vi "RootsPumpLCW_Main.vi"(7 "ref_stop_external":refnum<vi>, 8 "variable_reference":T1) -> ()   [LabVIEW 2019]
uses:
  cluster_ref_RootsPumpLCW.ctl
  <vilib>/MakerHub/LINX/LMH-LINX.lvlib
panel:
  out "time_now":dbl
  in  "Logging":bool=TRUE
  out "Logging Status":bool
  in  "Tab Control":enum32{"Flow Chart", "Raw Voltage Chart"}(tab)
  out "M1 Chart":waveform(dbl)[](graph)
  out "M2 Chart":waveform(dbl)[](graph)
  out "M3 Chart":waveform(dbl)[](graph)
  out "M4 Chart":waveform(dbl)[](graph)
  out "WFS1 Chart":waveform(dbl)[](graph)
  in  "SMS":bool=TRUE
  in  "M123_lo":dbl=0.3 caption="M1/M2/M3"
  in  "M123_lolo":dbl=0.2
  in  "WFS1_lo":dbl=1.3 caption="WFS1"
  in  "WFS1_lolo":dbl=1.2
  out "alarm_status":u32(colorbox) caption="Alarm Status"
  out "M1 Voltage Chart":waveform(dbl)[](graph)
  out "M2 Voltage Chart":waveform(dbl)[](graph)
  out "M3 Voltage Chart":waveform(dbl)[](graph)
  out "M4 Voltage Chart":waveform(dbl)[](graph)
  out "WFS1 Voltage Chart":waveform(dbl)[](graph)
  out "M1_V":dbl caption="V" format="%.2g"
  out "M4_V":dbl caption="V" format="%.2g"
  out "M3_V":dbl caption="V" format="%.2g"
  out "M2_V":dbl caption="V" format="%.2g"
  out "WFS1_V":dbl caption="V" format="%.2g"
  out "Meas. steps":i32
  in  "n_avg":i32=1000 caption="N of samples per meas."
  out "WFS1":dbl format="%.2g"
  in  "VISA":refnum<visa-resource-name>="COM25"
  out "M4":dbl format="%.2g"
  out "M3":dbl format="%.2g"
  in  "Meas. Interval":i32=30
  out "M2":dbl format="%.2g"
  out "M1":dbl format="%.2g"
  out "Readout Status":bool
  out "Last Measured":timestamp format="%<%Y-%m-%d %H:%M:%S>T"
  in  "Stop":bool
  # "Roots-Pump LCW Flow"
  # "sec"
  # "("
  # ")"
  # "("
  # ")"
  # "GPM"
  # "GPM"
  # "GPM"
  # "GPM"
  # "GPM"
  # "Warning:"
  # "GPM"
  # "Error:"
  # "GPM"
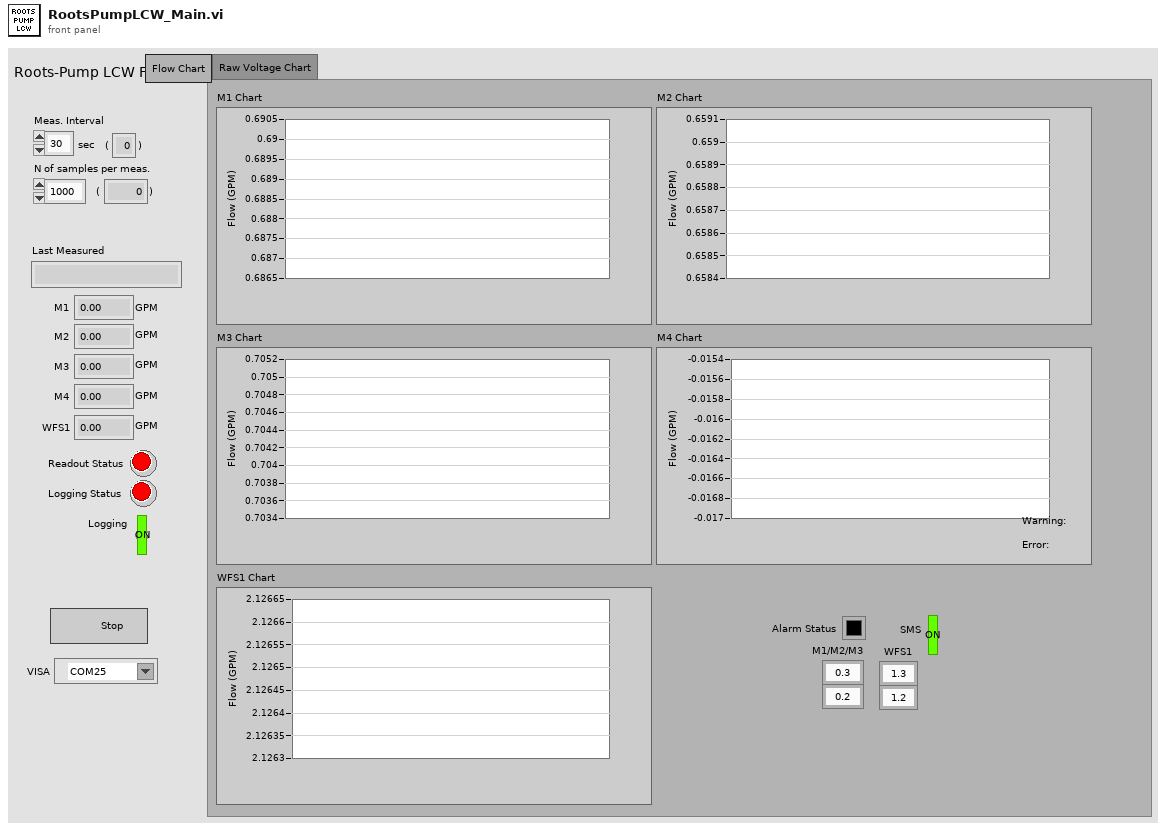
[diagram p1: front panel]
types:
  T1 = typedef "cluster_ref_RootsPumpLCW.ctl" = cluster{"Status":refnum<vi>, "M1":refnum<vi>, "M2":refnum<vi>, "M3":refnum<vi>, "M4":refnum<vi>, "WFS1":refnum<vi>}
  T2 = typedef "LMH-LINX.lvlib/LINX Ref.ctl" = cluster{"IO":T3, "Interface":T4, "LINX Device Config":T5}
  T3 = typedef "LMH-LINX.lvlib/Platform.ctl" = enum16{"Remote", "Local"}
  T4 = typedef "LMH-LINX.lvlib/Interface.ctl" = enum16{"Serial", "TCP"}
  T5 = typedef "LMH-LINX.lvlib/Device.lvlib/LINX Device Config.ctl" = cluster{"Interface":T4, "COM Port":refnum<visa-resource-name>, "TCP Configuration":T6, "Device Family":u8, "Device ID":u8, "Device Name":string, "TCP Ref":refnum<k5>, "Channels":T7}
  T6 = typedef "LMH-LINX.lvlib/Device.lvlib/TCP Config.ctl" = cluster{"IP Address":string, "Port":u16}
  T7 = typedef "LMH-LINX.lvlib/Channels.ctl" = cluster{"DI":u8[], "DO":u8[], "AI":u8[], "AO":u8[], "PWM":u8[], "QE":u8[], "UART":u8[], "I2C 2":u8[], "SPI":u8[], "CAN":u8[], "Servo":u8[], "AI Ref (V)":dbl, "AI Resolution (Bits)":u8, "AO Ref (V)":dbl, "AO Resolution (Bits)":u8}
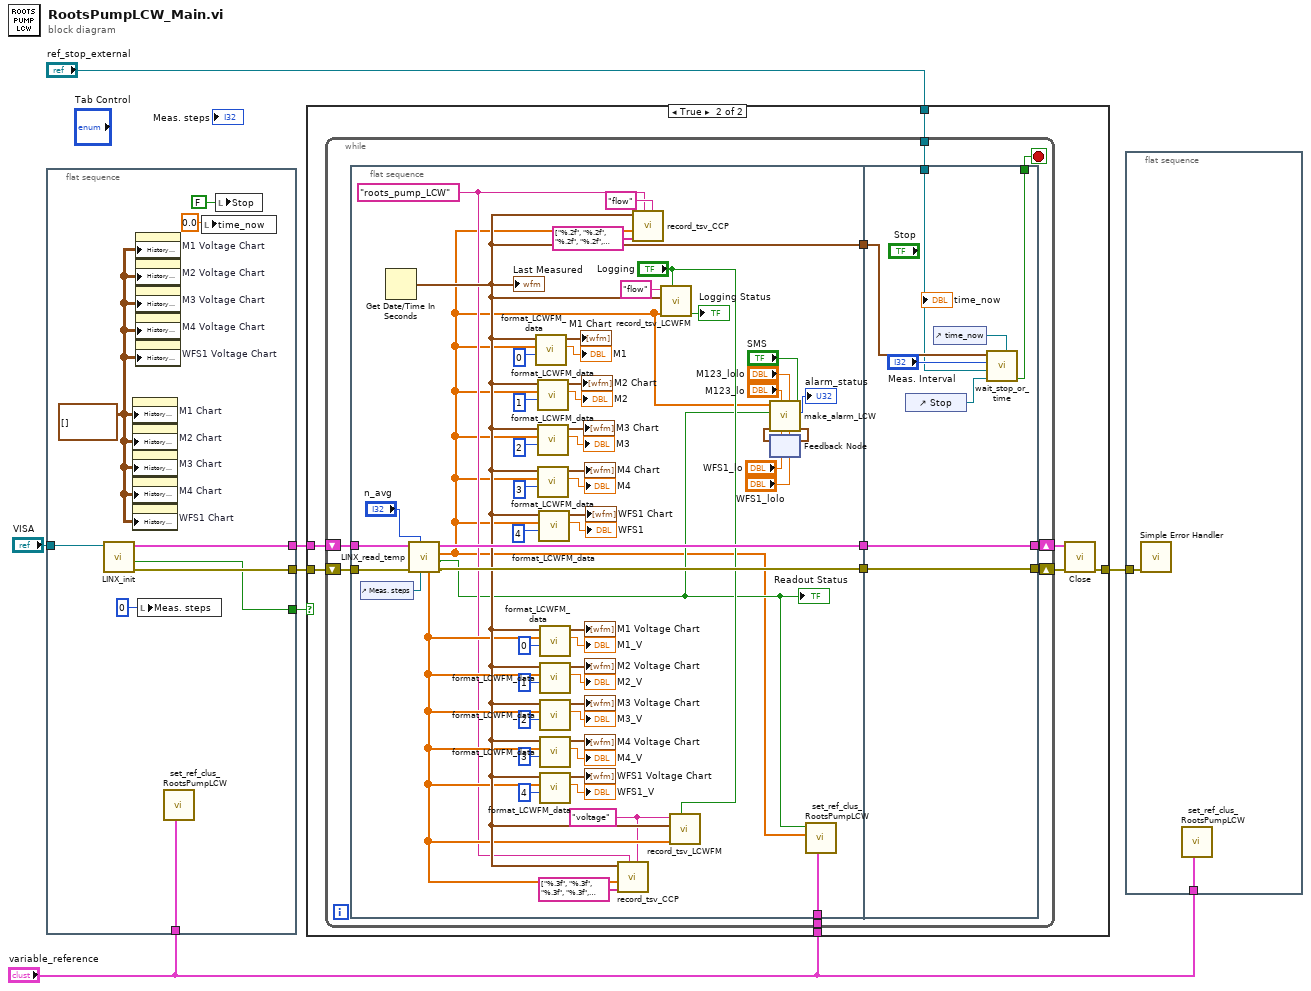
[diagram p0: block diagram]
diagram:
  n1 = flat-sequence {
    tunnel: [w13] -> w6
    tunnel: [w16] -> w5
    tunnel: "VISA" -> [w15]
    tunnel: [w14] -> w3
    tunnel: "variable_reference" -> [w8]
    frame #0 {
      w11 = waveform(dbl)[][] [] ("History Data")
      n2 = call "LINX_init.vi"("VISA"=w15) -> ("error out"=w16:errorcluster, "status"=w13:bool, "LINX Resource"=w14:T2)  [unwired: 8 in]
      n3 = property on="M1 Chart" class="WFChart (strict)"("History Data"=w11) -> ()  [unwired: 2 in, 2 out]
      n4 = property on="M2 Chart" class="WFChart (strict)"("History Data"=w11) -> ()  [unwired: 2 in, 2 out]
      n5 = property on="M3 Chart" class="WFChart (strict)"("History Data"=w11) -> ()  [unwired: 2 in, 2 out]
      n6 = property on="M4 Chart" class="WFChart (strict)"("History Data"=w11) -> ()  [unwired: 2 in, 2 out]
      n7 = property on="WFS1 Chart" class="WFChart (strict)"("History Data"=w11) -> ()  [unwired: 2 in, 2 out]
      n8 = property on="M1 Voltage Chart" class="WFChart (strict)"("History Data"=w11) -> ()  [unwired: 2 in, 2 out]
      n9 = property on="M2 Voltage Chart" class="WFChart (strict)"("History Data"=w11) -> ()  [unwired: 2 in, 2 out]
      n10 = property on="M3 Voltage Chart" class="WFChart (strict)"("History Data"=w11) -> ()  [unwired: 2 in, 2 out]
      n11 = property on="M4 Voltage Chart" class="WFChart (strict)"("History Data"=w11) -> ()  [unwired: 2 in, 2 out]
      n12 = property on="WFS1 Voltage Chart" class="WFChart (strict)"("History Data"=w11) -> ()  [unwired: 2 in, 2 out]
      n13 = local write "Meas. steps"(0 ("Meas. steps")) -> ()
      n14 = call "set_ref_clus_RootsPumpLCW.vi"("variable_reference"=w8) -> ()  [unwired: 11 in]
      n15 = local write "time_now"(0.0 ("time_now")) -> ()
      n16 = local write "Stop"(FALSE ("Stop")) -> ()
    }
  }
  n17 = case shown="True" w6 {
    tunnel: [w17 w22] -> w7
    tunnel: w5 -> [w17 w24]
    tunnel: w3 -> [_ w23]
    tunnel: "variable_reference" -> [_ w19]
    tunnel: "ref_stop_external" -> [_ w18]
    frame False {
    }
    frame True {
      n18 = while {
        shift-right: [w31] -> w21
        shift-left: w24 -> [w34]
        shift-right: [w32] -> w20
        shift-left: w23 -> [w33]
        tunnel: w19 -> [w26]
        tunnel: w18 -> [w25]
        stop <- w28 stop-if-true
        n19 = flat-sequence {
          tunnel: w34 -> [w88]
          tunnel: w33 -> [w87]
          tunnel: [w86] -> w30
          tunnel: [w85] -> w29
          tunnel: [w42] -> w27
          tunnel: w26 -> [w37]
          tunnel: [w98] -> w31
          tunnel: [w99] -> w32
          tunnel: w30 -> [w99]
          tunnel: w29 -> [w98]
          tunnel: [w95] -> w28
          tunnel: w27 -> [w97]
          tunnel: w25 -> [w92]
          frame #0 {
            w39 = "roots_pump_LCW" ("folder_name")
            w38 = "voltage" ("file_name")
            n20 = control-ref of="Meas. steps"() -> (w82:refnum<vi>)
            n21 = Get Date/Time In Seconds() -> (seconds since 1Jan1904=w42:timestamp)
            "Last Measured" <- w42
            n22 = call "LINX_read_temp.vi"("n_step"=w82, "n_avg"="n_avg", "Error In"=w88, "LINX Resource"=w87) -> ("Error Out"=w85:errorcluster, "status"=w36:bool, "array_flow"=w35:dbl[], "LINX Resource Out"=w86:T2, "array_voltage"=w41:dbl[])  [unwired: 3 in]
            "Readout Status" <- w36
            n23 = call "format_LCWFM_data.vi"("index"=0, "value_array"=w35, "time"=w42) -> ("value"=→"M1":dbl, "waveform_array"=→"M1 Chart":waveform(dbl)[])  [unwired: 7 in]
            n24 = call "format_LCWFM_data.vi"("index"=1, "value_array"=w35, "time"=w42) -> ("value"=→"M2":dbl, "waveform_array"=→"M2 Chart":waveform(dbl)[])  [unwired: 7 in]
            n25 = call "format_LCWFM_data.vi"("index"=2, "value_array"=w35, "time"=w42) -> ("value"=→"M3":dbl, "waveform_array"=→"M3 Chart":waveform(dbl)[])  [unwired: 7 in]
            n26 = call "format_LCWFM_data.vi"("index"=3, "value_array"=w35, "time"=w42) -> ("value"=→"M4":dbl, "waveform_array"=→"M4 Chart":waveform(dbl)[])  [unwired: 7 in]
            n27 = call "format_LCWFM_data.vi"("index"=4, "value_array"=w35, "time"=w42) -> ("value"=→"WFS1":dbl, "waveform_array"=→"WFS1 Chart":waveform(dbl)[])  [unwired: 7 in]
            n28 = call "format_LCWFM_data.vi"("index"=0, "value_array"=w41, "time"=w42) -> ("value"=→"M1_V":dbl, "waveform_array"=→"M1 Voltage Chart":waveform(dbl)[])  [unwired: 7 in]
            n29 = call "format_LCWFM_data.vi"("index"=1, "value_array"=w41, "time"=w42) -> ("value"=→"M2_V":dbl, "waveform_array"=→"M2 Voltage Chart":waveform(dbl)[])  [unwired: 7 in]
            n30 = call "format_LCWFM_data.vi"("index"=2, "value_array"=w41, "time"=w42) -> ("value"=→"M3_V":dbl, "waveform_array"=→"M3 Voltage Chart":waveform(dbl)[])  [unwired: 7 in]
            n31 = call "format_LCWFM_data.vi"("index"=3, "value_array"=w41, "time"=w42) -> ("value"=→"M4_V":dbl, "waveform_array"=→"M4 Voltage Chart":waveform(dbl)[])  [unwired: 7 in]
            n32 = call "format_LCWFM_data.vi"("index"=4, "value_array"=w41, "time"=w42) -> ("value"=→"WFS1_V":dbl, "waveform_array"=→"WFS1 Voltage Chart":waveform(dbl)[])  [unwired: 7 in]
            n33 = call "record_tsv_CCP.vi"("file_name"=w38, "folder_name"=w39, "format_array"=string[] ["%.3f", "%.3f", "%.3f", "%.3f", "%.3f"], "value_array"=w41, "time"=w42) -> ()  [unwired: 5 in, 2 out]
            n34 = call "record_tsv_CCP.vi"("file_name"="flow", "folder_name"=w39, "format_array"=string[] ["%.2f", "%.2f", "%.2f", "%.2f", "%.2f"], "value_array"=w35, "time"=w42) -> ()  [unwired: 5 in, 2 out]
            n35 = call "record_tsv_LCWFM.vi"("record_on"="Logging", "value_array"=w35, "time"=w42, "file_name"="flow") -> ("status"=→"Logging Status":bool)  [unwired: 7 in]
            n36 = call "record_tsv_LCWFM.vi"("record_on"="Logging", "value_array"=w41, "time"=w42, "file_name"=w38) -> ()  [unwired: 7 in, 1 out]
            n37 = feedback #1() -> (w47:timestamp)  [unwired: 1 in]
            n38 = call "make_alarm_LCW.vi"("enabled"="SMS", "WFS1_lolo"="WFS1_lolo", "M123_lolo"="M123_lolo", "WFS1_lo"="WFS1_lo", "M123_lo"="M123_lo", "time_last_alarm_in"=w47, "readout_status"=w36, "value_array"=w35) -> ("time_last_alarm_out"=w48:timestamp, "alarm_status"=→"alarm_status":u32)  [unwired: 2 in]
            n39 = feedback-in #1(w48) -> ()
            n40 = call "set_ref_clus_RootsPumpLCW.vi"("variable_reference"=w37, "array_flow"=w35, "status"=w36) -> ()  [unwired: 9 in]
          }
          frame #1 {
            n41 = control-ref of="Stop"() -> (w93:refnum<vi>)
            n42 = control-ref of="time_now"() -> (w94:refnum<vi>)
            n43 = call "wait_stop_or_time.vi"("ref_time_remain"=w94, "ref_stop_internal"=w93, "ref_stop_external"=w92, "time_wait"="Meas. Interval", "time0"=w97) -> ("stop_out"=w95:bool)  [unwired: 6 in]
          }
        }
      }
      n44 = call <vilib>:"Close.vi"("Error In"=w21, "LINX Resource"=w20) -> ("Error Out"=w22:errorcluster)  [unwired: 9 in]
    }
  }
  n45 = flat-sequence {
    tunnel: w7 -> [w101]
    tunnel: "variable_reference" -> [w100]
    frame #0 {
      n46 = call <vilib>:"Simple Error Handler.vi"("error in (no error)"=w101) -> ()  [unwired: 4 in, 5 out]
      n47 = call "set_ref_clus_RootsPumpLCW.vi"("variable_reference"=w100) -> ()  [unwired: 11 in]
    }
  }
